vi "Engine Init.vi"(6 "Device Reference":T3 format="%.0x", 8 "error in (no error)":errorcluster, 9 "Notifier in":refnum<notifier>, 10 "Device Inputs FIFO":refnum<k33>, 11 "Device Outputs FIFO":refnum<k33>) -> (0 "error out":errorcluster, 3 "Engine Run-Time Data Cluster":T1 {"Compiled Data"."Corruption Info DUT_Network"."Frame Infos Array"."CRC Index" min=-7 max=7; "Compiled Data"."Corruption Info DUT_Network"."Frame Infos Array"."DLC Length  Corruption Index" min=-8 max=8; "Compiled Data"."Corruption Info Network_DUT"."Frame Infos Array"."CRC Index" min=-7 max=7; "Compiled Data"."Corruption Info Network_DUT"."Frame Infos Array"."DLC Length  Corruption Index" min=-8 max=8; "Specified Channel Ref List Out" format="%.0x"; "Specified Channel Ref List In" format="%.0x"})   [LabVIEW 2018, in "CAN Gateway Engine.lvlib"]
uses:
  CAN Gateway Engine.lvlib
  <vilib>/NI Veristand/Custom Device API/Custom Device Item Ref.ctl
  Shared/CTLs/Runtime engine Data.ctl
  <vilib>/NI Veristand/Custom Device API/Custom Device Engine Event Ref.ctl
  Shared/CTLs/Compiled Data.ctl
  Shared/CTLs/Corruption Info.ctl
  Shared/CTLs/Frame.ctl
  Shared/CTLs/Signal_Data_Trigger.ctl
  <vilib>/NI Veristand/Custom Device API/Custom Device Channel Type.ctl
  Shared/Constants.vi
  <vilib>/NI Veristand/Custom Device API/Get Item Property (Variant).vi
  <vilib>/NI Veristand/Custom Device API/Custom Device API.lvlib
  <vilib>/NI Veristand/Custom Device Tools/Custom Device Utility Library/Custom Device Utility Library.lvlib
  Shared/CAN Gateway Shared.lvlib
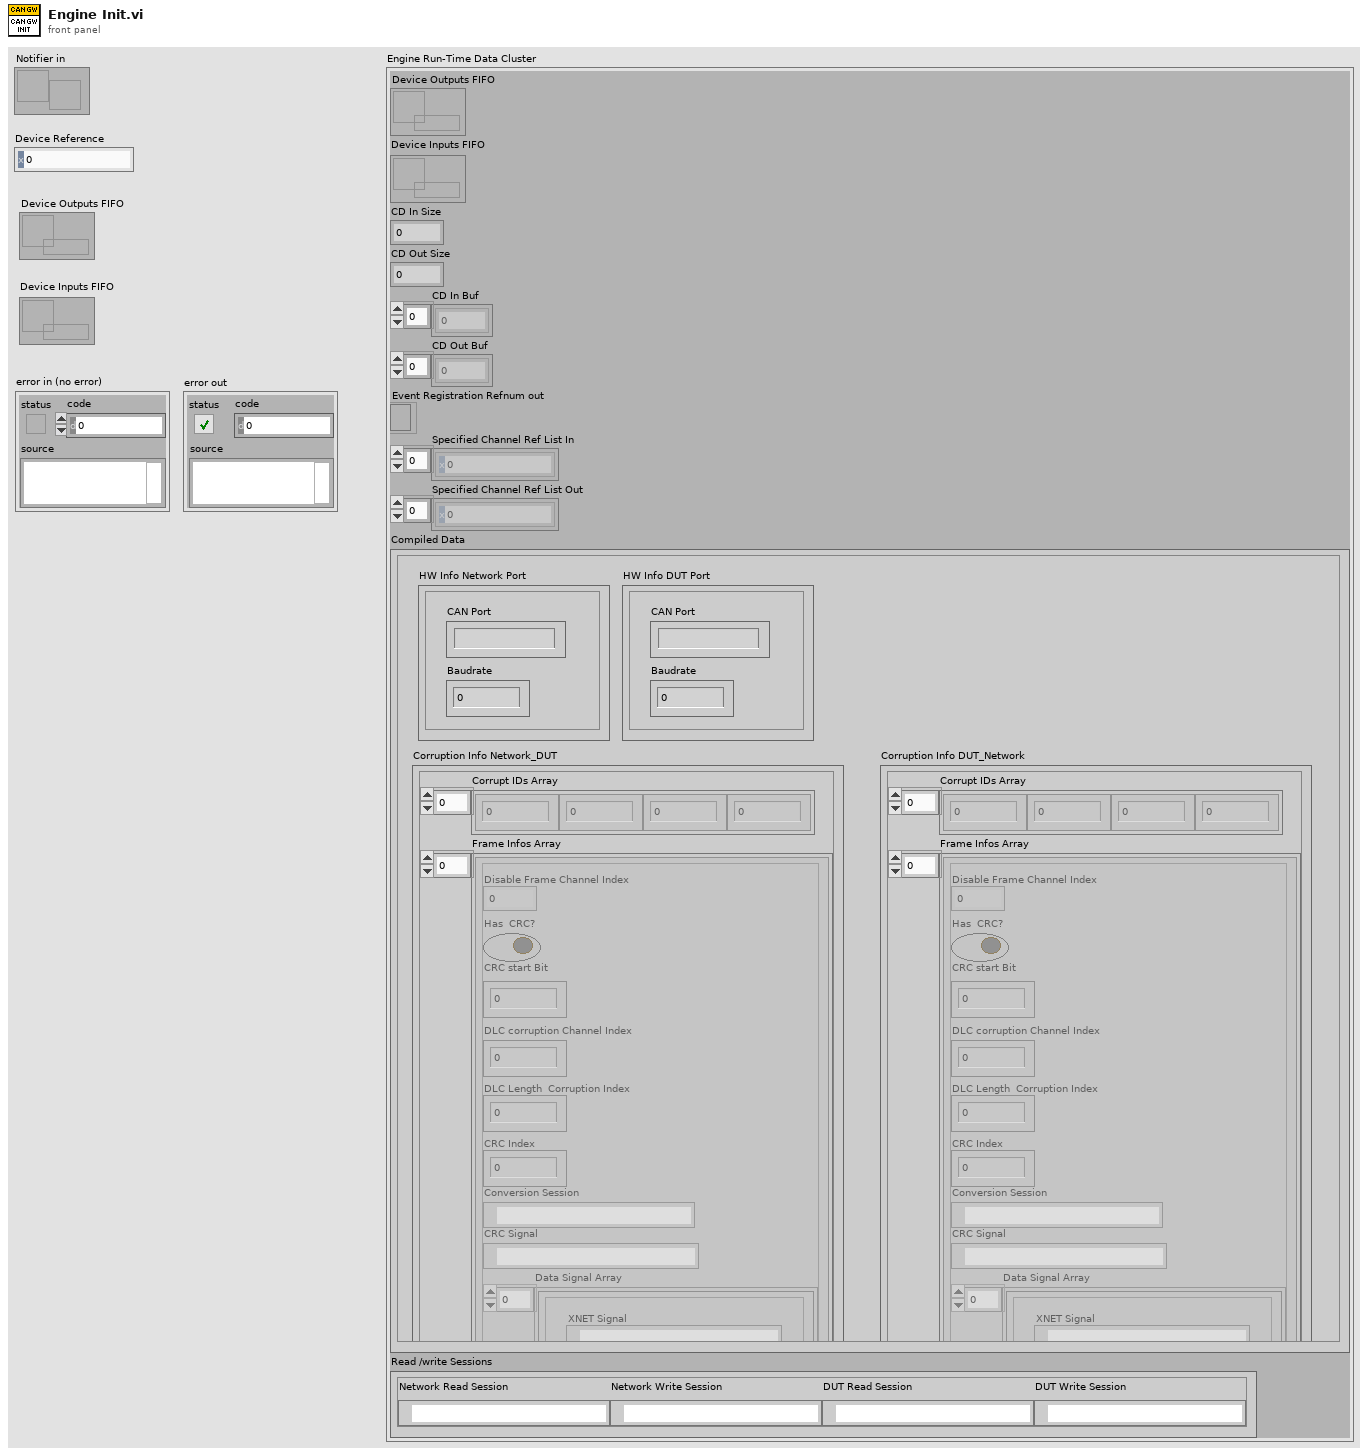
[diagram p1: front panel]
types:
  T1 = typedef "CAN Gateway Engine.lvlib/Runtime engine Data.ctl" = cluster{"Device Outputs FIFO":refnum<k33>, "Device Inputs FIFO":refnum<k33>, "CD In Size":i32, "CD Out Size":i32, "CD In Buf":dbl[], "CD Out Buf":dbl[], "Event Registration Refnum out":T2, "Specified Channel Ref List In":T3[], "Specified Channel Ref List Out":T3[], "Compiled Data":T4, "Read /write Sessions":cluster{"Network Read Session":refnum<k21>, "Network Write Session":refnum<k21>, "DUT Read Session":refnum<k21>, "DUT Write Session":refnum<k21>}}
  T2 = typedef "Custom Device API.lvlib/Custom Device Engine Event Ref.ctl" = refnum<event-registration>
  T3 = typedef "Custom Device API.lvlib/Custom Device Item Ref.ctl" = u64
  T4 = typedef "CAN Gateway Shared.lvlib/Compiled Data.ctl" = cluster{"HW Info Network Port":cluster{"CAN Port":string, "Baudrate":u64}, "HW Info DUT Port":cluster{"CAN Port":string, "Baudrate":u64}, "Corruption Info Network_DUT":T5, "Corruption Info DUT_Network":T5}
  T5 = typedef "CAN Gateway Shared.lvlib/Corruption Info.ctl" = cluster{"Corrupt IDs Array":u32[], "Frame Infos Array":T6[]}
  T6 = typedef "CAN Gateway Shared.lvlib/Frame.ctl" = cluster{"Disable Frame Channel Index":i32, "Has  CRC?":bool, "CRC start Bit":u32, "DLC corruption Channel Index":i32, "DLC Length  Corruption Index":i32, "CRC Index":i32, "Conversion Session":refnum<k21>, "CRC Signal":refnum<k21>, "Data Signal Array":T7[]}
  T7 = typedef "CAN Gateway Shared.lvlib/Signal_Data_Trigger.ctl" = cluster{"XNET Signal":refnum<k21>, "Data Idx":u32, "Trigger Idx":u32}
  T8 = typedef "Custom Device API.lvlib/Custom Device Channel Type.ctl" = enum16{"Input", "Output"}
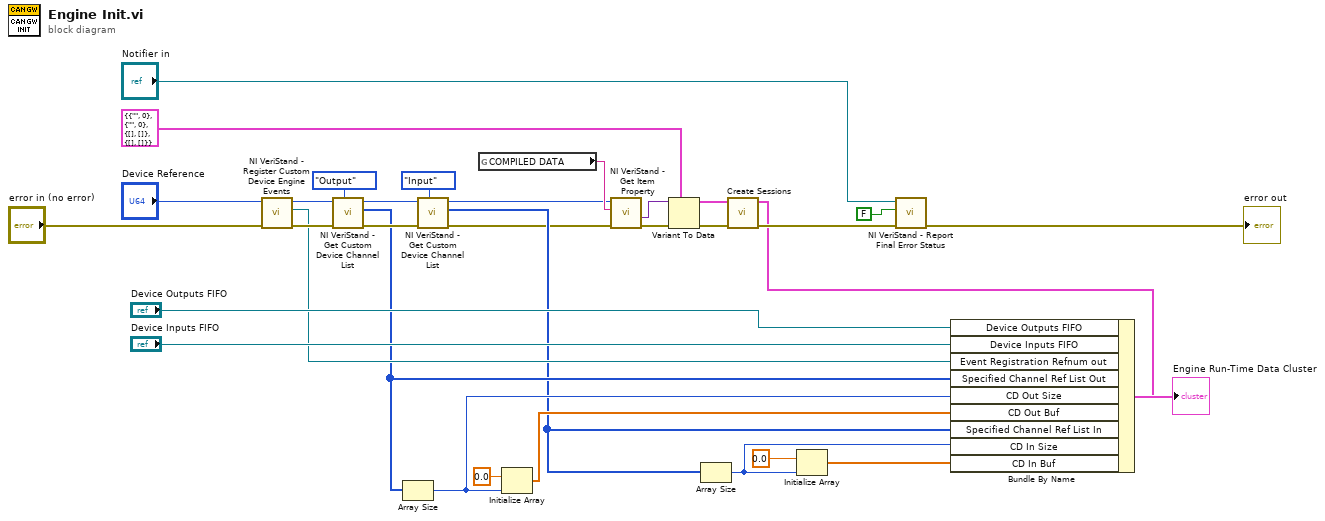
[diagram p0: block diagram]
diagram:
  n1 = call <vilib>:"NI VeriStand - Register Custom Device Engine Events.vi"("error in (no error)"="error in (no error)", "Device Ref in"="Device Reference") -> ("error out"=w23:errorcluster, "Custom Device Engine Event Ref"=w20:T2, "Device Ref out"=w30:T3)  [unwired: 7 in]
  n2 = call <vilib>:"NI VeriStand - Get Custom Device Channel List.vi"("Channel Type"=Custom_Device_Channel_Type."Output", "error in (no error)"=w23, "Device Ref in"=w30) -> ("error out"=w27:errorcluster, "Specified Channel Ref List"=w19:T3[], "Device Ref out"=w26:T3)  [unwired: 6 out]
  n3 = Array Size(array=w19) -> (size(s)=w18:i32)
  n4 = call <vilib>:"NI VeriStand - Get Custom Device Channel List.vi"("Channel Type"=Custom_Device_Channel_Type."Input", "error in (no error)"=w27, "Device Ref in"=w26) -> ("error out"=w9:errorcluster, "Specified Channel Ref List"=w16:T3[], "Device Ref out"=w3:T3)  [unwired: 6 out]
  n5 = global read "Constants.vi" "COMPILED DATA"() -> (w7:string)
  n6 = Initialize Array(0.0 ("element"), w18) -> (w17:dbl[])
  n7 = call-poly <vilib>:"NI VeriStand - Get Item Property.vi"("error in (no error)"=w9, "Property Name"=w7, "Item Ref in"=w3) -> ("error out"=w8:errorcluster, "Value"=w4:variant)  [unwired: 5 in, 2 out]
  n8 = Variant To Data(error in=w8, type=T4 {"HW Info Network Port"={"CAN Port"="", "Baudrate"=0}, "HW Info DUT Port"={"CAN Port"="", "Baudrate"=0}, "Corruption Info Network_DUT"={"Corrupt IDs Array"=[], "Frame Infos Array"=[]}, "Corruption Info DUT_Network"={"Corrupt IDs Array"=[], "Frame Infos Array"=[]}} ("Compiled Data"), Variant=w4) -> (data=w1:T4, error out=w6:errorcluster)
  n9 = Array Size(array=w16) -> (size(s)=w15:i32)
  n10 = call "Create Sessions.vi"("error in (no error)"=w6, "Compiled Data in"=w1) -> ("error out"=w12:errorcluster, "Engine Run-Time Data Cluster"=w10:T1)  [unwired: 8 in]
  n11 = Initialize Array(0.0 ("element"), w15) -> (w14:dbl[])
  n12 = call <vilib>:"NI VeriStand - Report Final Error Status.vi"("error in (no error)"=w12, "Filter FIFO & Shutdown Errors (T)"=FALSE ("Filter FIFO Errors (T)"), "Status Notifier"="Notifier in") -> ("error out"=→"error out":errorcluster)  [unwired: 8 out]
  n13 = Bundle By Name(cluster=w10, "Device Outputs FIFO"="Device Outputs FIFO", "Device Inputs FIFO"="Device Inputs FIFO", "Event Registration Refnum out"=w20, "Specified Channel Ref List Out"=w19, "CD Out Size"=w18, "CD Out Buf"=w17, "Specified Channel Ref List In"=w16, "CD In Size"=w15, "CD In Buf"=w14) -> (→"Engine Run-Time Data Cluster":T1)
